vi "PrimaryAttackerRole.vi"(7 "firstCall":bool=TRUE, 8 "error in (no error)":errorcluster, 10 "Game in":refnum<class "Game.lvclass">, 11 "PrimaryAttackerRole_v2 in":refnum<class "PrimaryAttackerRole_v2.lvclass">) -> (0 "error out":errorcluster, 1 "Game out":refnum<class "Game.lvclass">, 2 "Robot out":refnum<class "Robot.lvclass">, 3 "PrimaryAttackerRole_v2 out":refnum<class "PrimaryAttackerRole_v2.lvclass">)   [LabVIEW 2023, in "PrimaryAttackerRole_v2.lvclass"]
uses:
  PrimaryAttackerRole_v2.lvclass
  C:/Users/ebert/Documents/codes/SSL/repo/SSL_AI/Role_class/Role.lvclass
  Game_class/Game.lvclass
  Robot_class/Robot.lvclass
  Role_class/Role.lvclass/Role.ctl
  Game_class/Game.lvclass/Game.ctl
  Object_class/Object.lvclass/Object.ctl
  Robot_class/Robot.lvclass/Robot.ctl
  Game_class/Read BallRef.vi
  Object_class/Read x.vi
  Object_class/Read y.vi
  Robot_class/Write dest_x.vi
  Robot_class/Write dest_y.vi
  Robot_class/Write dest_orientation.vi
  Role_class/Read Tacticbook.vi
  Role_class/Write tactic_index.vi
  Role_class/Write Tacticbook.vi
  Role_class/Read RobotRef.vi
  Ball_class/Ball.lvclass
  C:/Users/ebert/Documents/codes/SSL/repo/SSL_AI/Object_class/Object.lvclass
  Tacticbook_class/Tacticbook.lvclass
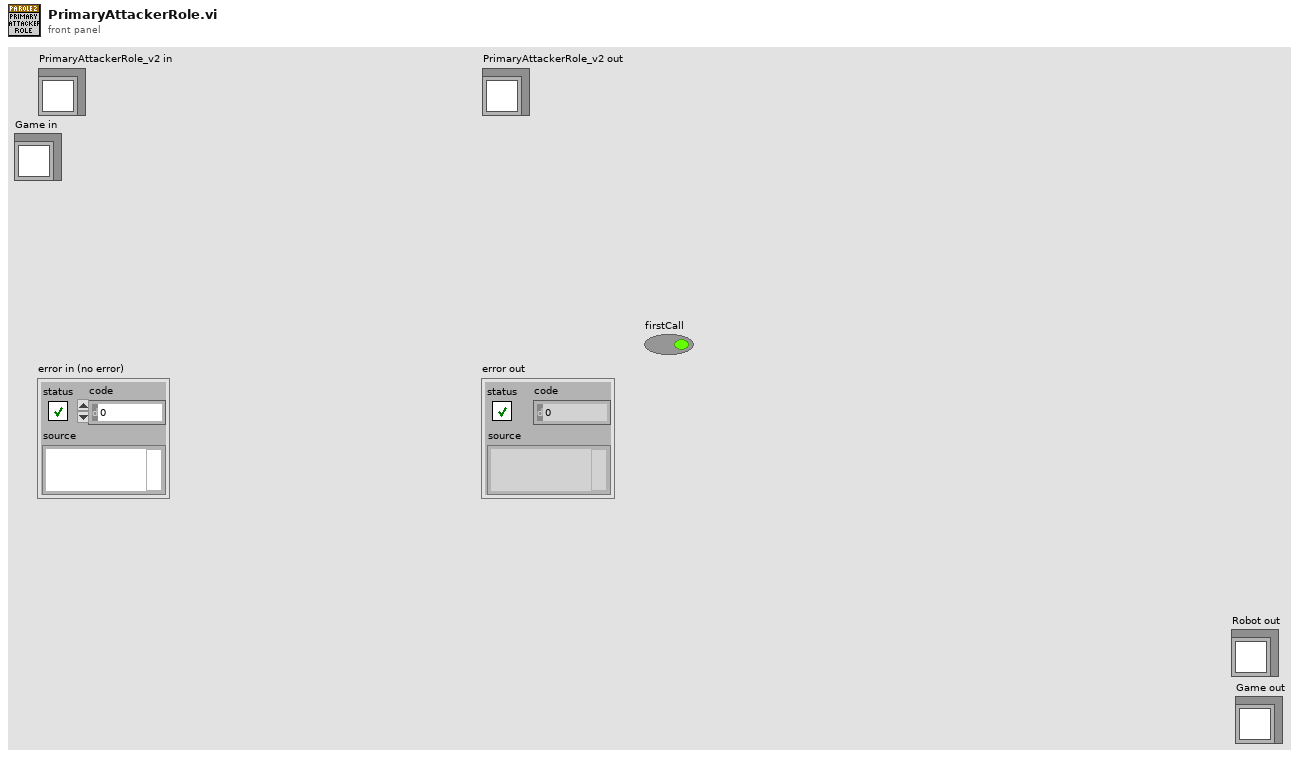
[diagram p1: front panel]
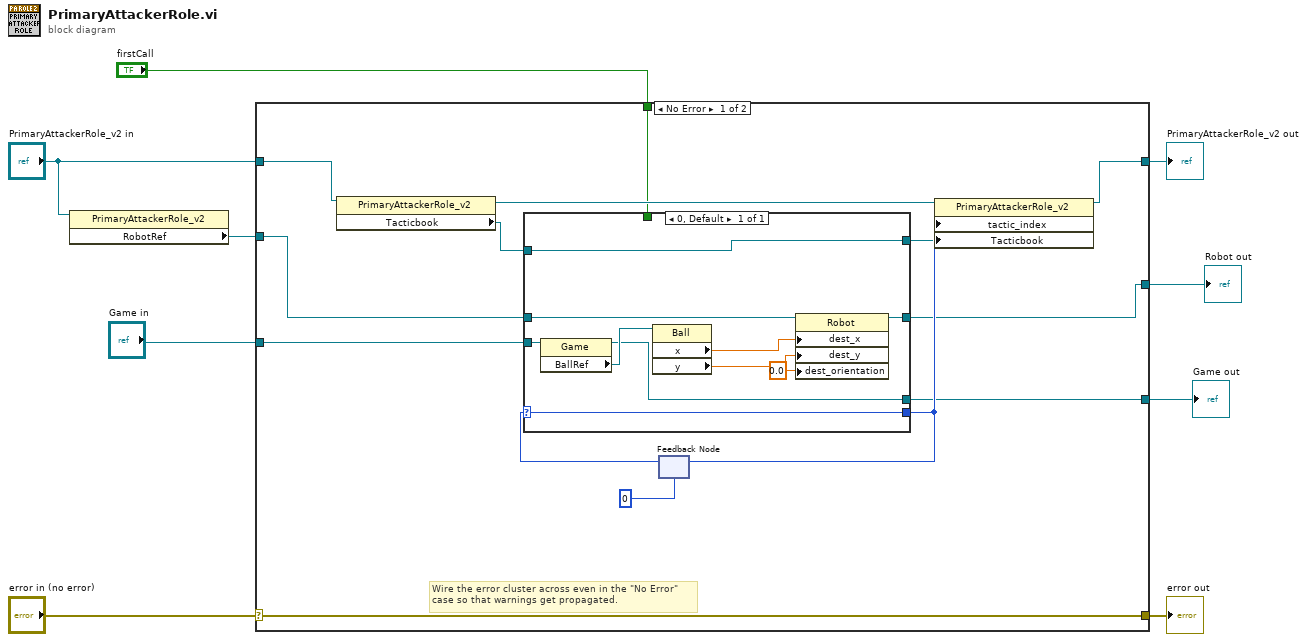
[diagram p0: block diagram]
diagram:
  n1 = property class="PrimaryAttackerRole_v2"(reference="PrimaryAttackerRole_v2 in") -> ("RobotRef"=w4:refnum<class "Robot.lvclass">)  [unwired: 1 in, 2 out]
  n2 = case shown="No Error" "error in (no error)" {
    selector: "error in (no error)" -> [w23 w37]
    tunnel: [w23 w37] -> w8
    tunnel: [w17 w36] -> w7
    tunnel: "PrimaryAttackerRole_v2 in" -> [w16 w36]
    tunnel: "Game in" -> [w14 w34]
    tunnel: w4 -> [w15 w35]
    tunnel: [w10 w35] -> w3
    tunnel: [w11 w34] -> w2
    tunnel: "firstCall" -> [w13 _]
    frame No Error {
      # "Wire the error cluster across even in the \"No Error\"\ncase so that warnings get propagated."
      n3 = property class="PrimaryAttackerRole_v2"(reference=w16) -> (reference out=w22:refnum<class "PrimaryAttackerRole_v2.lvclass">, "Tacticbook"=w19:refnum<class "Tacticbook.lvclass">)  [unwired: 1 in, 1 out]
      n4 = feedback #1(0) -> (w20:i32)
      n5 = case shown="0, Default" w20 {
        selector: w20 -> [w33]
        tunnel: [w33] -> w18
        tunnel: w19 -> [w26]
        tunnel: w15 -> [w30]
        tunnel: w14 -> [w32]
        tunnel: w13 -> [_]
        tunnel: [w26] -> w12
        tunnel: [w25] -> w11
        tunnel: [w24] -> w10
        frame 0, Default {
          n6 = property class="Game"(reference=w32) -> (reference out=w25:refnum<class "Game.lvclass">, "BallRef"=w31:refnum<class "Ball.lvclass">)  [unwired: 1 in, 1 out]
          n7 = property class="Ball"(reference=w31) -> ("x"=w29:dbl, "y"=w28:dbl)  [unwired: 1 in, 2 out]
          n8 = property class="Robot"(reference=w30, "dest_x"=w29, "dest_y"=w28, "dest_orientation"=0.0) -> (reference out=w24:refnum<class "Robot.lvclass">)  [unwired: 1 in, 1 out]
        }
      }
      n9 = feedback-in #1(w18) -> ()
      n10 = property class="PrimaryAttackerRole_v2"(reference=w22, "tactic_index"=w18, "Tacticbook"=w12) -> (reference out=w17:refnum<class "PrimaryAttackerRole_v2.lvclass">)  [unwired: 1 in, 1 out]
    }
    frame Error {
    }
  }
  "error out" <- w8
  "PrimaryAttackerRole_v2 out" <- w7
  "Robot out" <- w3
  "Game out" <- w2
